vi "OP150ZP_Param_ConfZENplusOP100.vi"(8 "errin":errorcluster, 10 "Chaîne":string, 11 "pathin":path) -> (0 "errout":errorcluster, 3 "VISA OUT":cluster{"BT3562":string})   [LabVIEW 2020]
uses:
  <vilib>/Utility/config.llb/Read Key (String).vi
  <vilib>/Utility/config.llb/NI_LVConfig.lvlib
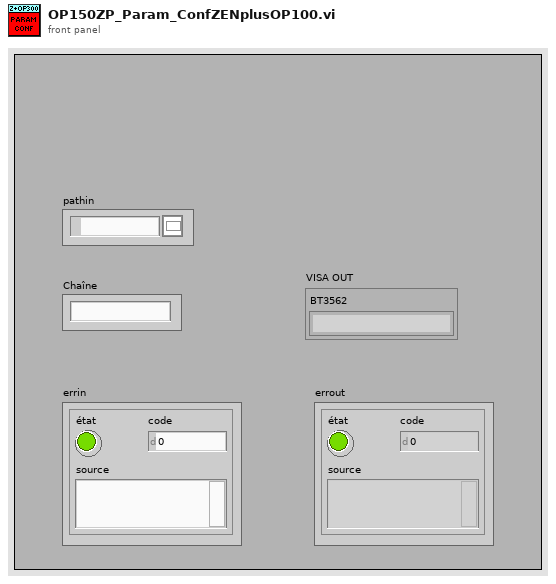
[diagram p1: front panel]
types:
  T1 = typedef "NI_LVConfig.lvlib/Config Data RefNum.ctl" = refnum<k1>
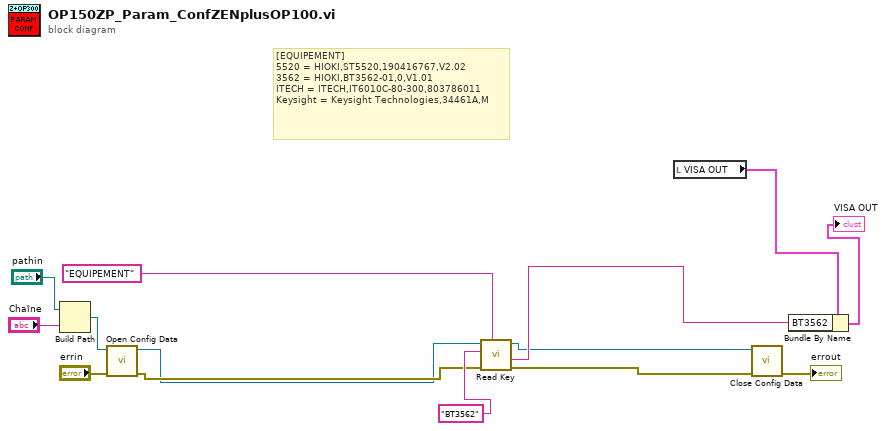
[diagram p0: block diagram]
diagram:
  # "[EQUIPEMENT]\n5520 = HIOKI,ST5520,190416767,V2.02\n3562 = HIOKI,BT3562-01,0,V1.01\nITECH = ITECH,IT6010C-80-300,803786011\nKeysight = Keysight Technologies,34461A,M"
  n1 = Build Path(base path="pathin", name or relative path="Chaîne") -> (appended path=w13:path)
  n2 = call <vilib>:"Open Config Data.vi"("error in (no error)"="errin", "configuration file path"=w13) -> ("error out"=w2:errorcluster, "refnum"=w1:T1)  [unwired: 7 in, 1 out]
  n3 = call-poly <vilib>:"Read Key.vi"("section"="EQUIPEMENT", "error in (no error)"=w2, "key"="BT3562", "refnum"=w1) -> ("error out"=w4:errorcluster, "value"=w7:string, "refnum out"=w3:T1)  [unwired: 4 in, 1 out]
  n4 = local read "VISA OUT"() -> (w9:cluster{"BT3562":string})
  n5 = call <vilib>:"Close Config Data.vi"("error in (no error)"=w4, "refnum"=w3) -> ("error out"=→"errout":errorcluster)  [unwired: 8 in, 1 out]
  n6 = Bundle By Name(cluster=w9, "BT3562"=w7) -> (→"VISA OUT":cluster{"BT3562":string})
